vi "Robot Global Data.vi"() -> ()   [LabVIEW 2013]
doc: "This global VI can contain as many global variables as you need. Place a control on the panel, give it a good name. To read or write to it from a VI, drag the icon to the diagram of that VI. You can also drag from the project. Click on the node to change which global you access. You shouldn't have multiple locations writing to a global or it will cause a race-condition."
uses:
  <vilib>/Rock Robotics/WPI/Camera/WPI_CameraImageSize.ctl
  <vilib>/Rock Robotics/WPI/DriverStation/WPI_DriverStationRobotMode2.ctl
panel:
  in  "cToggleArcade":bool
  in  "cDirection":dbl
  in  "cThrottle":dbl
  in  "IsArcade?":bool
  in  "cElevatedPass":bool
  in  "cGroundPass":bool
  in  "cServo":dbl
  in  "cClapperIn":bool
  in  "cClapperOut":bool
  in  "cPass":bool
  in  "cAutoDistance":bool
  in  "cCatch":bool
  in  "cCollectorWrap":bool
  in  "cHandleSolenoid":bool
  in  "cKickerPneumatic":bool
  in  "cFiringPneumatic":bool
  in  "cRollerPneumatic":bool
  in  "cCollector":dbl
  in  "cRoller":dbl
  in  "cShooter":bool
  in  "cReverseDrive":bool
  in  "cSonicShifter":bool
  in  "cStraightDrive":bool
  in  "cHalfDrive":bool
  in  "cTankDriveRight":dbl
  in  "cTankDriveLeft":dbl
  in  "Robot Mode":T1
  in  "LED toggle rate (ms)":u32=20
  in  "image size":T2=enum."320x240"
  in  "Enable Vision":bool
  # "MISC"
  # "VISION"
  # "DRIVE"
  # "ROLLER"
  # "WRAPPERS"
  # "Collector"
  # "Pneumatics"
  # "DRIVER"
  # "SHOOTER"
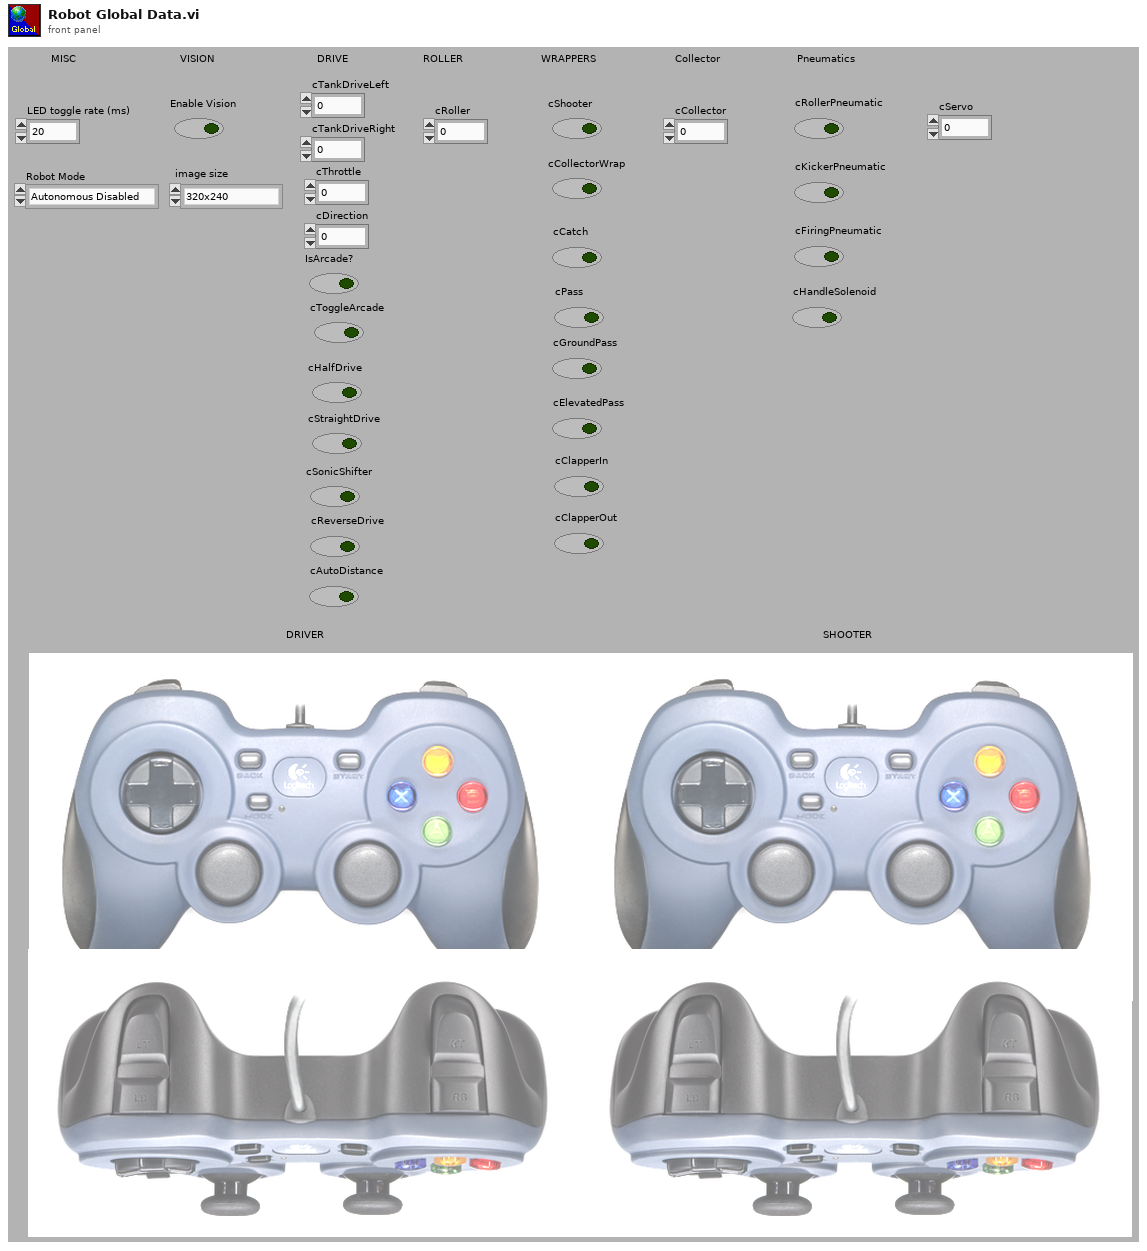
[diagram p1: front panel]
types:
  T1 = typedef "WPI_DriverStationRobotMode2.ctl" = enum16{"Autonomous Disabled", "Autonomous Enabled", "Teleop Disabled", "Teleop Enabled", "Timeout", "Finish", "Test Disabled", "Test Enabled"}
  T2 = typedef "WPI_CameraImageSize.ctl" = enum16{"640x480", "320x240", "160x120"}
diagram:
